vi "analysis.vi"() -> ()   [LabVIEW 2018, in "analysis.lvlib"]
uses:
  analysis.lvlib
panel:
  out "Array":dbl[](array[numeric])
  in  "Numeric":i32
  in  "Samples":i32=4000
  out "Waveform Graph":dynamicdata(graph)
  in  "Data":enum16{"191122", "191123", "200410", ""}(ring)
  out "Filename Out":path
  out "Error":errorcluster
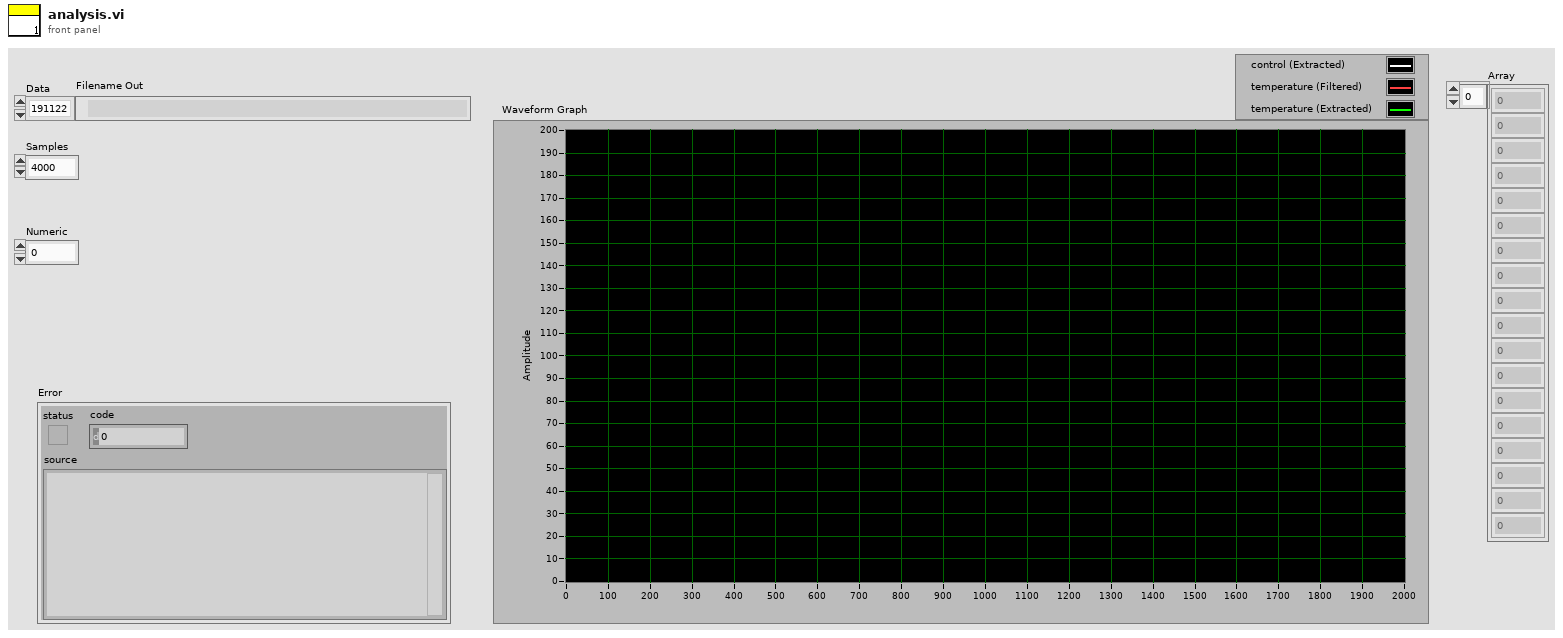
[diagram p1: front panel]
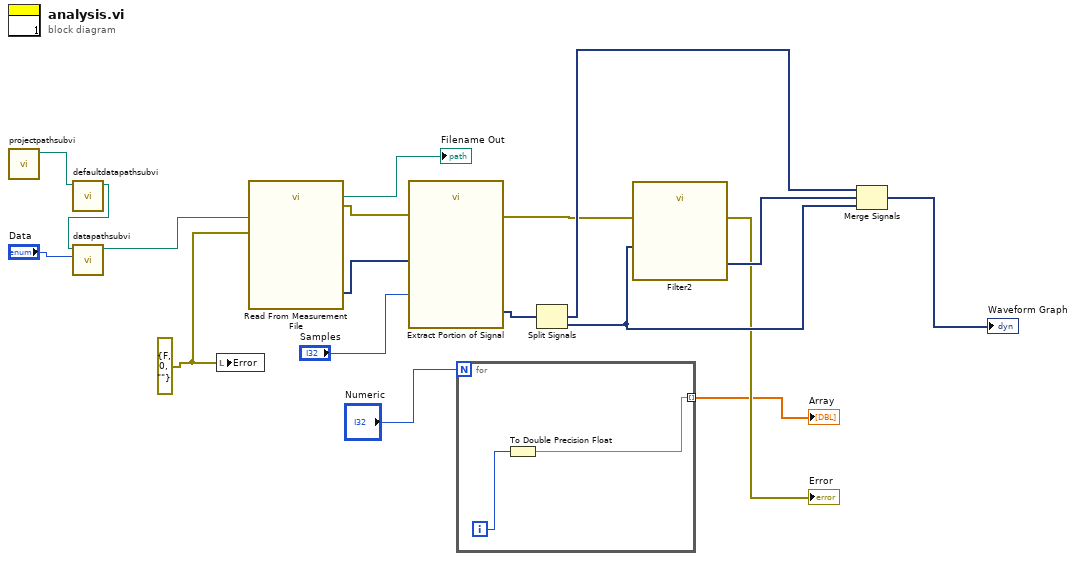
[diagram p0: block diagram]
diagram:
  w17 = errorcluster {"status"=FALSE, "code"=0, "source"=""} ("File Error")
  n1 = call "projectpathsubvi.vi"() -> ("stripped path"=w13:path)  [unwired: 11 in]
  n2 = call "defaultdatapathsubvi.vi"("stripped path"=w13) -> ("default data path"=w14:path)  [unwired: 10 in]
  n3 = call "datapathsubvi.vi"("Data"="Data", "default data path"=w14) -> ("appended path"=w12:path)  [unwired: 9 in]
  n4 = local write "Error"(w17) -> ()
  n5 = call "Read From Measurement File"("error in (no error)"=w17, "Filename"=w12) -> ("error out"=w10:errorcluster, "Filename Out"=→"Filename Out":path, "Signals"=w9:dynamicdata)  [unwired: 4 in, 3 out]
  n6 = call "Extract Portion of Signal"("error in (no error)"=w10, "Samples"="Samples", "Signals"=w9) -> ("error out"=w6:errorcluster, "Section"=w7:dynamicdata)  [unwired: 7 in]
  n7 = for {
    N: "Numeric" -> [_]
    tunnel: [w20] -> w1 mode=indexing
    i -> [w19]
    n8 = To Double Precision Float(number=w19) -> (double precision float=w20:dbl)
  }
  "Array" <- w1
  n9 = Split Signals(w7) -> (w18:dynamicdata, w4:dynamicdata)  [unwired: 3 in, 1 out]
  n10 = call "Filter2"("error in (no error)"=w6, "Signal"=w4) -> ("error out"=→"Error":errorcluster, "Filtered Signal"=w5:dynamicdata)  [unwired: 8 in]
  n11 = Merge Signals(w18, w5, w4) -> (→"Waveform Graph":dynamicdata)
